vi "Link Channel Core.vi"(8 "error in (no error)":errorcluster, 10 "Channel Connection":T1, 11 "CIF_UI in":refnum<class "CIF_UI.lvclass">) -> (0 "error out":errorcluster, 3 "CIF_UI out":refnum<class "CIF_UI.lvclass">)   [LabVIEW 2021, in "CIF_UI.lvclass"]
uses:
  CIF_UI.lvclass
  CIF_UI.lvclass/CIF_UI.ctl
  CIFCore/Grpc/CIFCoreChannel_client/RPC Messages/cif_channelcore_ConnectSubscriber.ctl
  CIFCore/Grpc/CIFCoreChannel_client/CIFCoreChannel_client.lvlib
  CIFCore/Common/CIFCoreCommon.lvlib
  CIFCore/Common/Typedef/Errors.ctl
  CIFCore/Grpc/CIFCoreWrapper/CIFCoreWrapper.lvlib
  CIFCore/Grpc/CIFCoreChannel_client/RPC Messages/cif_channelcore_ChannelPattern.ctl
  <vilib>/CIF Foundation/CIF Channels Core/ChannelCommon/typedef/New FIFO Instance Configuration.ctl
  <vilib>/CIF Foundation/CIF Channels Core/ChannelCommon/ChannelCommon.lvlib
  CIFCore/Common/Typedef/FIFO Publisher.ctl
  Typedef/Channel Connection.ctl
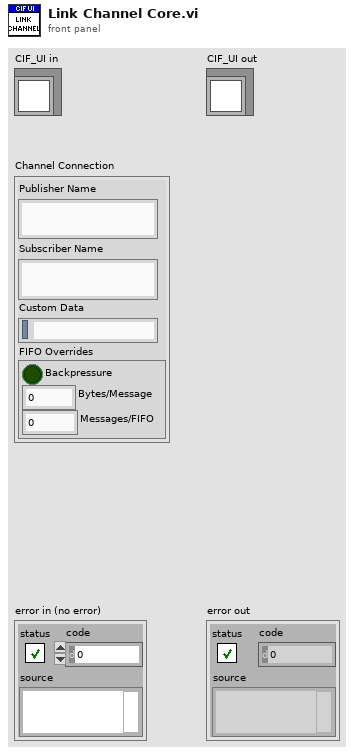
[diagram p1: front panel]
types:
  T1 = typedef "CIF_UI.lvclass/Channel Connection.ctl" = cluster{"Publisher Name":string, "Subscriber Name":string, "Custom Data":string, "FIFO Overrides":cluster{"Backpressure":bool, "Bytes/Message":u32, "Messages/FIFO":u32}}
  T2 = typedef "CIFCoreChannel_client.lvlib/cif_channelcore_ConnectSubscriber.ctl" = cluster{"subscriber_name":string, "publisher_name":string, "custom_connect":u8[]}
  T3 = typedef "CIFCoreChannel_client.lvlib/cif_channelcore_Channel.ctl" = cluster{"name":string, "direction":T4, "type":string, "custom_config":u8[], "connected":bool, "connected_name":string, "forced":bool, "channel_pattern":T5}
  T4 = typedef "CIFCoreChannel_client.lvlib/cif_channelcore_ChannelDirection.ctl" = enum32{"CHANNELDIRECTION_UNKNOWN", "CHANNELDIRECTION_PUBLISHER", "CHANNELDIRECTION_SUBSCRIBER"}
  T5 = typedef "CIFCoreChannel_client.lvlib/cif_channelcore_ChannelPattern.ctl" = enum32{"CHANNELPATTERN_UNKNOWN", "CHANNELPATTERN_TAG", "CHANNELPATTERN_FIFO", "CHANNELPATTERN_MULTIFIFO", "CHANNELPATTERN_BACKPRESSUREFIFO"}
  T6 = typedef "CIFCoreCommon.lvlib/FIFO Publisher.ctl" = cluster{"Publisher Name":string, "New FIFO Instance Config":T7}
  T7 = typedef "ChannelCommon.lvlib/New FIFO Instance Configuration.ctl" = cluster{"Backpressure":bool, "Bytes/Message Override":u32, "Messages/FIFO Override":u32, "Custom Data":u8[]}
  T8 = typedef "CIFCoreCommon.lvlib/Errors.ctl" = enum16{"Invalid Clock ID", "Long Sleep", "gRPC Server Not Found", "Config Parse", "Timestamp Wrap", "Delayed Execution", "Duplicate Channel", "Missing Channel", "Incorrect Type", "Flatten Error", "Unflatten Data", "Unique Name", "Plugin Not Found", "Plugin Type Not Found", "Plugin Version Not Found", "Manager Not Found", "Numerical Issue", "Time Jump", "Clock ID Match", "Channel Length", "Plugin Connection", "gRPC Server Connection", "PPL Name Match", "Build", "Config Log Parse", "Plugin Load", "UI Subpanel Load", "Python Name", "Invalid Name", "Unable to Change Ch Buffer"}
  T9 = typedef "CIF_UI.lvclass/Plugin Connection Map.ctl" = map{string, T10}
  T10 = typedef "CIF_UI.lvclass/Plugin Connections.ctl" = cluster{"gRPC ID":T11, "Plugin Info":T12}
  T11 = typedef "grpc-lvsupport-release.lvlib/grpcId.ctl" = u64
  T12 = typedef "CIF_UI.lvclass/PluginInfo.ctl" = cluster{"Name":string, "Type":string, "grpc_port":i32, "Version":T13, "Node Status":T14}
  T13 = typedef "CIF_UI.lvclass/Version.ctl" = cluster{"Major":i32, "Minor":i32, "Fix":i32}
  T14 = typedef "CIFCoreCommon.lvlib/gRPC Reported Plugin Status.ctl" = cluster{"State":T15, "Timing Statistics (us)":T16, "FIFO Statistics (us)":T18, "error":T19, "Monitor Doubles":T20, "Monitor U64":T21, "Monitor I64":T22}
  T15 = typedef "CIFCoreCommon.lvlib/Plugin State.ctl" = enum32{"Null", "Creating", "Listening", "Running", "CleaningUp", "Destroying"}
  T16 = typedef "CIFCoreCommon.lvlib/Timing Statistics.ctl" = cluster{"Period":T17, "Wake Error":T17, "Execute":T17, "Housekeep":T17, "Idle":T17, "Cleanup":T17, "Custom 1 (custom units)":T17, "Custom 2 (custom units)":T17}
  T17 = typedef "CIFCoreCommon.lvlib/Timing Stats Base.ctl" = cluster{"Max":i64, "Avg":dbl, "Min":i64}
  T18 = typedef "CIFCoreCommon.lvlib/FIFO Statistics.ctl" = cluster{"From T0":T17, "From Previous Plugin":T17, "Output Error":T17}
  T19 = typedef "CIFCoreCommon.lvlib/Simple Error.ctl" = cluster{"status":bool, "code":i32}
  T20 = typedef "CIFCoreCommon.lvlib/Monitor Doubles.ctl" = cluster{"1":dbl, "2":dbl, "3":dbl, "4":dbl}
  T21 = typedef "CIFCoreCommon.lvlib/Monitor U64.ctl" = cluster{"1":u64, "2":u64, "3":u64, "4":u64}
  T22 = typedef "CIFCoreCommon.lvlib/Monitor I64.ctl" = cluster{"1":i64, "2":i64, "3":i64, "4":i64}
  T23 = typedef "ChannelCommon.lvlib/New FIFO Instance Response.ctl" = cluster{"Publisher":string, "Custom Data":u8[]}
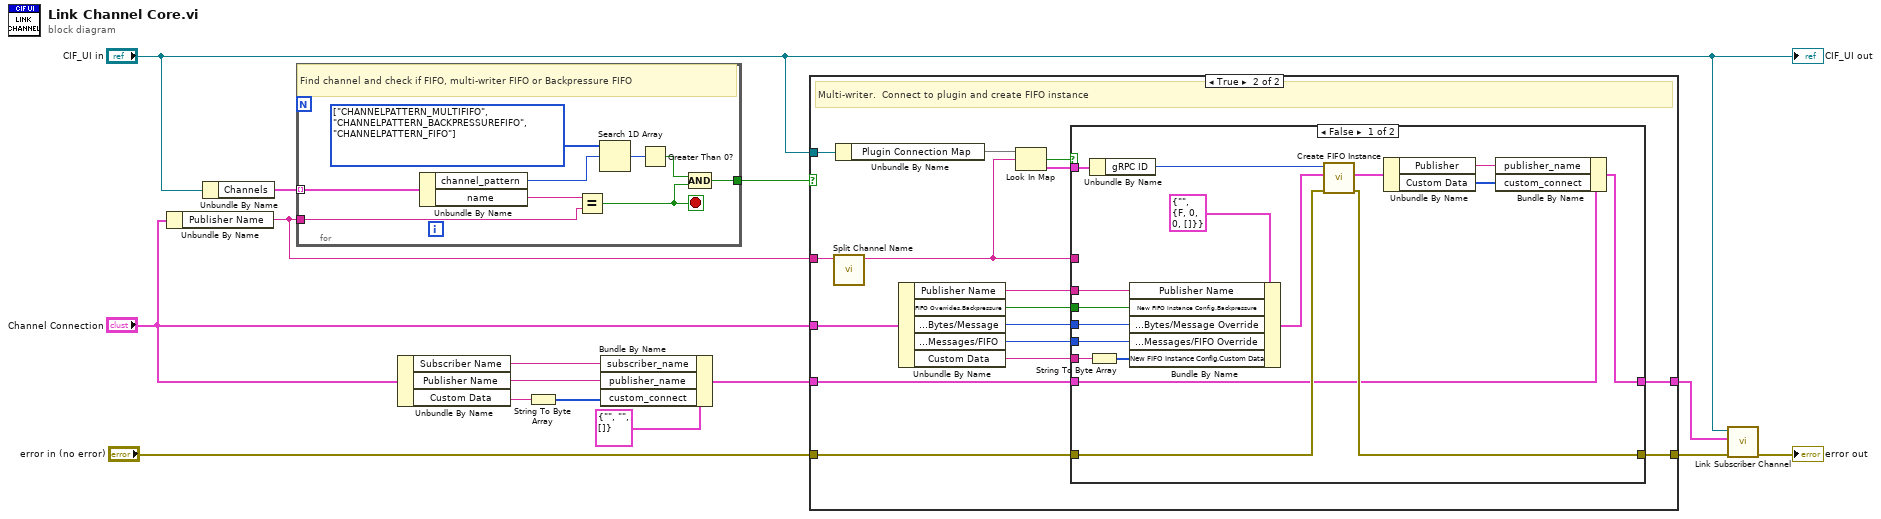
[diagram p0: block diagram]
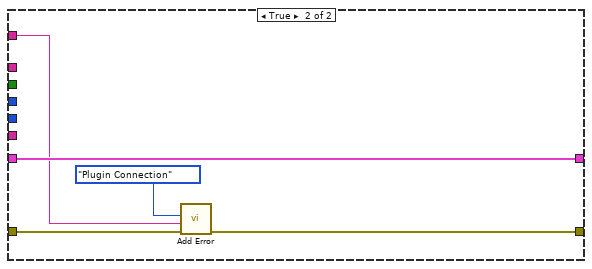
[diagram p3: hidden frame]
diagram:
  n1 = Unbundle By Name("Channel Connection") -> ("Publisher Name"=w14:string)
  n2 = Unbundle By Name("CIF_UI in") -> ("Channels"=w15:T3[])
  n3 = for {
    tunnel: w15 -> [w24] mode=indexing
    tunnel: [w21] -> w13
    tunnel: w14 -> [w20]
    stop <- w22 stop-if-true
    w19 = T5[] [enum."CHANNELPATTERN_MULTIFIFO", enum."CHANNELPATTERN_BACKPRESSUREFIFO", enum."CHANNELPATTERN_FIFO"] items=["CHANNELPATTERN_UNKNOWN", "CHANNELPATTERN_TAG", "CHANNELPATTERN_FIFO", "CHANNELPATTERN_MULTIFIFO", "CHANNELPATTERN_BACKPRESSUREFIFO"] ("1D array")
    # "Find channel and check if FIFO, multi-writer FIFO or Backpressure FIFO"
    n4 = Unbundle By Name(w24) -> ("channel_pattern"=w18:T5, "name"=w23:string)
    n5 = Equal?(x=w23, y=w20) -> (x = y?=w22:bool)
    n6 = Search 1D Array(1D array=w19, element=w18) -> (index of element=w17:i32)  [unwired: 1 in]
    n7 = Greater Than 0?(x=w17) -> (x > 0?=w16:bool)
    n8 = Compound Arithmetic op=AND(w16, w22) -> (w21:bool)
  }
  n9 = Unbundle By Name("Channel Connection") -> ("Subscriber Name"=w9:string, "Publisher Name"=w8:string, "Custom Data"=w7:string)
  n10 = String To Byte Array(string=w7) -> (unsigned byte array=w11:u8[])
  n11 = Bundle By Name(cluster=T2 {"subscriber_name"="", "publisher_name"="", "custom_connect"=[]} ("Connection 2"), "subscriber_name"=w9, "publisher_name"=w8, "custom_connect"=w11) -> (w5:T2)
  n12 = case shown="True" w13 {
    tunnel: w14 -> [_ w29]
    tunnel: "CIF_UI in" -> [_ w41]
    tunnel: "error in (no error)" -> [w25 w38]
    tunnel: "Channel Connection" -> [_ w37]
    tunnel: w5 -> [w26 w32]
    tunnel: [w26 w31] -> w3
    tunnel: [w25 w30] -> w4
    frame False {
      # "Not a multi-writer FIFO.  No need to contact publisher."
    }
    frame True {
      # "Multi-writer.  Connect to plugin and create FIFO instance"
      n13 = call "Split Channel Name.vi"("Channel Name"=w29) -> ("Parent"=w28:string)  [unwired: 8 in, 2 out]
      n14 = Unbundle By Name(w41) -> ("Plugin Connection Map"=w42:T9)
      n15 = Unbundle By Name(w37) -> ("Publisher Name"=w36:string, "FIFO Overrides.Backpressure"=w35:bool, "FIFO Overrides.Bytes/Message"=w34:u32, "FIFO Overrides.Messages/FIFO"=w33:u32, "Custom Data"=w27:string)
      n16 = Look In Map(map=w42, key=w28) -> (key not found?=w40:bool, value=w39:T10)  [unwired: 1 in]
      n17 = case shown="False" w40 {
        tunnel: w39 -> [w59 _]
        tunnel: [w58 w62] -> w30
        tunnel: w38 -> [w56 w63]
        tunnel: w28 -> [_ w61]
        tunnel: w36 -> [w55 _]
        tunnel: w35 -> [w54 _]
        tunnel: w34 -> [w53 _]
        tunnel: w33 -> [w52 _]
        tunnel: w32 -> [w51 w64]
        tunnel: [w50 w64] -> w31
        tunnel: w27 -> [w44 _]
        frame False {
          n18 = String To Byte Array(string=w44) -> (unsigned byte array=w43:u8[])
          n19 = Unbundle By Name(w59) -> ("gRPC ID"=w57:T11)
          n20 = Bundle By Name(cluster=T6 {"Publisher Name"="", "New FIFO Instance Config"={"Backpressure"=FALSE, "Bytes/Message Override"=0, "Messages/FIFO Override"=0, "Custom Data"=[]}} ("New Publisher"), "Publisher Name"=w55, "New FIFO Instance Config.Backpressure"=w54, "New FIFO Instance Config.Bytes/Message Override"=w53, "New FIFO Instance Config.Messages/FIFO Override"=w52, "New FIFO Instance Config.Custom Data"=w43) -> (w48:T6)
          n21 = call "Create FIFO Instance.vi"("error in"=w56, "New Publisher"=w48, "gRPC ID"=w57) -> ("error out"=w58:errorcluster, "FIFO Instance"=w47:T23)  [unwired: 6 in, 1 out]
          n22 = Unbundle By Name(w47) -> ("Publisher"=w46:string, "Custom Data"=w45:u8[])
          n23 = Bundle By Name(cluster=w51, "publisher_name"=w46, "custom_connect"=w45) -> (w50:T2)
        }
        frame True {
          n24 = call "Add Error.vi"("error in (no error)"=w63, "String to Append"=w61, "Error"=Errors."Plugin Connection") -> ("error out"=w62:errorcluster)  [unwired: 8 in]
        }
      }
    }
  }
  n25 = call "Link Subscriber Channel.vi"("error in (no error)"=w4, "Connection"=w3, "CIF_UI in"="CIF_UI in") -> ("error out"=→"error out":errorcluster)  [unwired: 8 in]
  "CIF_UI out" <- "CIF_UI in"
